vi "ExReadGenericFile.vi"() -> ()   [LabVIEW 2010]
panel:
  in  "Data Type":T1(ring)
  in  "Full File Name":path
  in  "Swap Bytes":bool
  in  "Header Size (Bytes)":u32
  in  "Z Dimension( Number of Frames)":u32=1
  in  "Y Dimension":u32
  in  "X Dimension":u32
  in  "?":bool
  out "error out":errorcluster
  in  "error in (no error)":errorcluster
  # "NOTICE\n\nTHIS VI REQUIRES THAT THE TOOLKIT\nBE UNLOADED BY RUNNING THE\n VI EXCLOSEGLOBALCAM.VI\n BEFORE LEAVING LABVIEW."
  # "ExReadGenericFile.vi\nThis VI will allow the user to read and display an image from a generic data file in which a header of known size is followed by one or more images of the same size.  The user must know the size of the header in bytes, the X/Y dimensions of an image, the number of images, the type of data and if byte swapping is required.\nWhen using this VI, be sure to hit the CLOSE IMAGE button when finished viewing the image.  This allows the image to be closed and the memory deallocated properly."
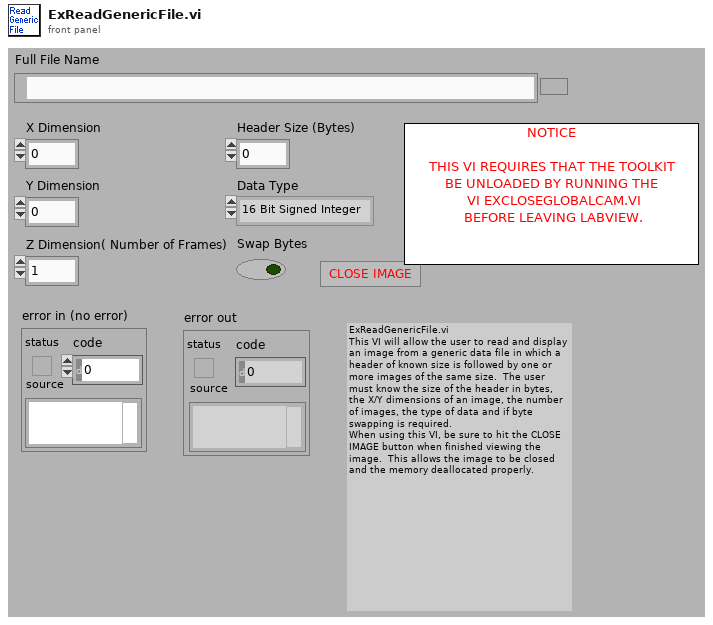
[diagram p1: front panel]
types:
  T1 = enum16{"16 Bit Signed Integer", "16 Bit Unsigned Integer", "32 Bit Signed Integer", "32 Bit Unsigned Integer", "8 Bit Signed Integer", "8 Bit Unsigned Integer", "32 Bit Floating Point", "64 Bit Floating Point"}
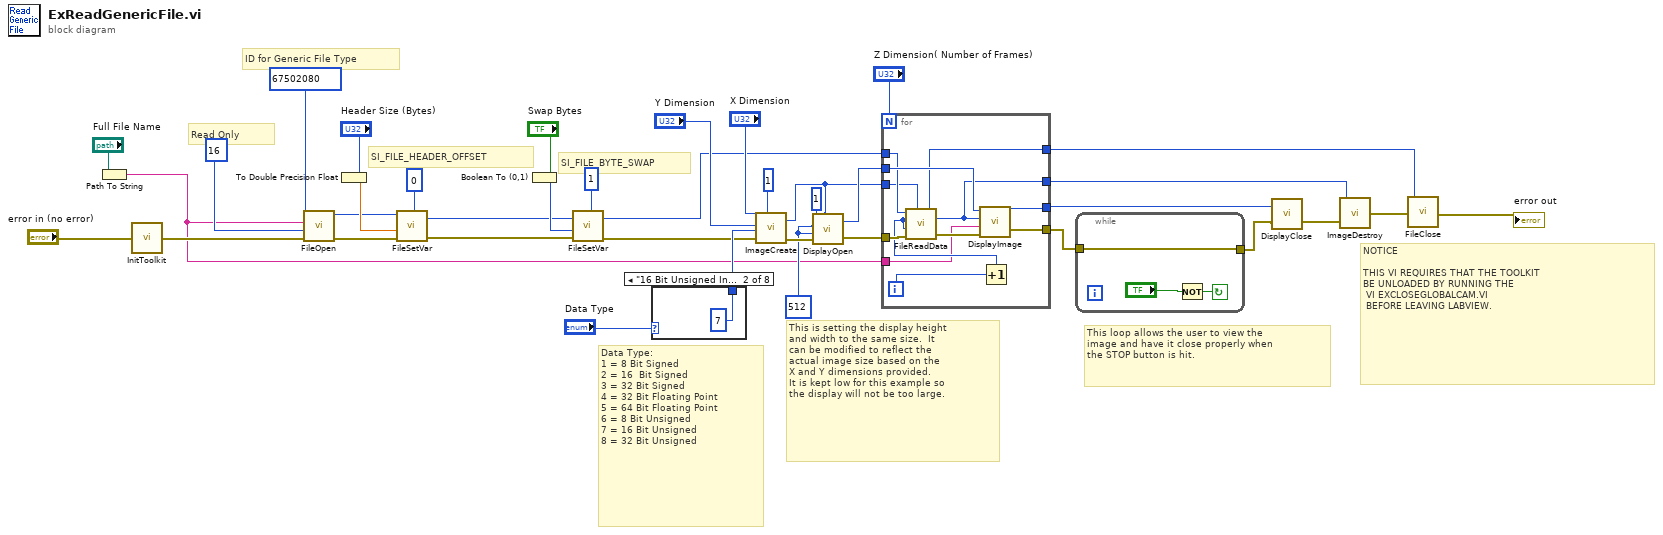
[diagram p0: block diagram]
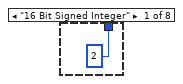
[diagram p2: hidden frame]
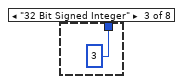
[diagram p3: hidden frame]
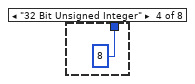
[diagram p4: hidden frame]
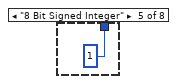
[diagram p5: hidden frame]
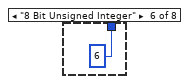
[diagram p6: hidden frame]
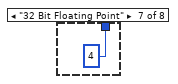
[diagram p7: hidden frame]
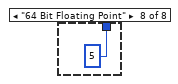
[diagram p8: hidden frame]
diagram:
  w35 = 512
  # "NOTICE\n\nTHIS VI REQUIRES THAT THE TOOLKIT\nBE UNLOADED BY RUNNING THE\n VI EXCLOSEGLOBALCAM.VI\n BEFORE LEAVING LABVIEW."
  # "This loop allows the user to view the \nimage and have it close properly when\nthe STOP button is hit."
  # "This is setting the display height \nand width to the same size.  It \ncan be modified to reflect the\nactual image size based on the\nX and Y dimensions provided.\nIt is kept low for this example so\nthe display will not be too large."
  # "Data Type:\n1 = 8 Bit Signed\n2 = 16  Bit Signed\n3 = 32 Bit Signed\n4 = 32 Bit Floating Point\n5 = 64 Bit Floating Point\n6 = 8 Bit Unsigned\n7 = 16 Bit Unsigned\n8 = 32 Bit Unsigned"
  # "SI_FILE_BYTE_SWAP"
  # "SI_FILE_HEADER_OFFSET"
  # "ID for Generic File Type"
  # "Read Only"
  n1 = Path To String(path="Full File Name") -> (string=w17:string)
  n2 = call <userlib>:"InitToolkit.vi"("error in"="error in (no error)") -> ("error out"=w38:errorcluster)
  n3 = call <userlib>:"FileOpen.vi"("error in"=w38, "File Operations"=16, "FileName"=w17, "File Type"=67502080) -> ("error out"=w16:errorcluster, "File Handle"=w5:u32)
  n4 = To Double Precision Float(number="Header Size (Bytes)") -> (double precision float=w11:dbl)
  n5 = call <userlib>:"FileSetVar.vi"("error in"=w16, "Value"=w11, "Parameter ID"=0, "File Handle"=w5) -> ("error out"=w15:errorcluster, "File Handle"=w3:u32)
  n6 = Boolean To (0,1)(Boolean="Swap Bytes") -> (0, 1=w9:i16)
  n7 = call <userlib>:"FileSetVar.vi"("error in"=w15, "Value"=w9, "Parameter ID"=1, "File Handle"=w3) -> ("error out"=w14:errorcluster, "File Handle"=w13:u32)
  n8 = case shown="\"16 Bit Unsigned Integer\"" "Data Type" {
    tunnel: [2 7 3 8 1 6 4 5] -> w18
    frame "16 Bit Signed Integer" {
    }
    frame "16 Bit Unsigned Integer" {
    }
    frame "32 Bit Signed Integer" {
    }
    frame "32 Bit Unsigned Integer" {
    }
    frame "8 Bit Signed Integer" {
    }
    frame "8 Bit Unsigned Integer" {
    }
    frame "32 Bit Floating Point" {
    }
    frame "64 Bit Floating Point" {
    }
  }
  n9 = call <userlib>:"ImageCreate.vi"("X dimension"="X Dimension", "Y dimension"="Y Dimension", "Data Type"=w18, "error in"=w14, "Number Of Frames"=1) -> ("Image Handle"=w31:u32, "error out"=w36:errorcluster)
  n10 = call <userlib>:"DisplayOpen.vi"("Image Handle"=w31, "error in"=w36, "Display Height"=w35, "Display Width"=w35, "Display Type"=1) -> ("error out"=w33:errorcluster, "Display Handle"=w32:u32)  [unwired: 1 in]
  n11 = for {
    N: "Z Dimension( Number of Frames)" -> [_]
    tunnel: w33 -> [w58]
    tunnel: w32 -> [w56]
    tunnel: w13 -> [w55]
    tunnel: w31 -> [w54]
    tunnel: [w51] -> w24
    tunnel: [w50] -> w30
    tunnel: [w49] -> w29
    tunnel: [w48] -> w26
    tunnel: w17 -> [w47]
    i -> [w53]
    n12 = Increment(x=w53) -> (x+1=w52:i32)
    n13 = call <userlib>:"FileReadData.vi"("File Handle"=w55, "Start Frame"=w52, "End Frame"=w52, "error in"=w58, "Image Handle"=w54) -> ("File Handle"=w49:u32, "Image Handle"=w48:u32, "error out"=w57:errorcluster)
    n14 = call <userlib>:"DisplayImage.vi"("error in"=w57, "Title"=w47, "Image Handle"=w48, "Display Handle"=w56) -> ("error out"=w51:errorcluster, "Display Handle"=w50:u32)
  }
  n15 = while {
    tunnel: w24 -> [w61]
    tunnel: [w61] -> w25
    stop <- w59 continue-if-true
    n16 = Not(x="?") -> (.not. x?=w59:bool)
  }
  n17 = call <userlib>:"DisplayClose.vi"("error in"=w25, "Display Handle"=w30) -> ("error out"=w28:errorcluster)
  n18 = call <userlib>:"ImageDestroy.vi"("error in"=w28, "Data handle"=w26) -> ("error out"=w27:errorcluster)
  n19 = call <userlib>:"FileClose.vi"("error in"=w27, "File Handle"=w29) -> ("error out"=→"error out":errorcluster)
